vi "BRig_dataExp_I_L_nTrig_PerState.vi"() -> (2 "output_I_L_nTrig_PerState":i32)   [LabVIEW 2014]
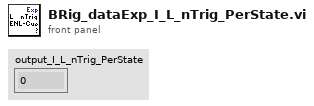
[diagram p1: front panel]
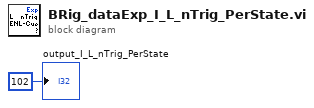
[diagram p0: block diagram]
diagram:
  "output_I_L_nTrig_PerState" <- 102 ("output_iBlock")
